vi "GetCellStrColor.vi"(7 "Color":u32, 8 "error in (no error)":errorcluster, 10 "Hdr Name":T1, 11 "Dynamic in":refnum<class "Dynamic.lvclass">) -> (0 "error out":errorcluster, 1 "Cell String":string, 2 "Cell Color":u32, 3 "Dynamic out":refnum<class "Dynamic.lvclass">)   [LabVIEW 2018, in "Measurement Channels.lvlib" / "Dynamic.lvclass"]
uses:
  Dynamic.lvclass
  Common/Controls/HeaderNames.ctl
  Dynamic.lvclass/Dynamic.ctl
  SubVIs Table/Custom Ctls Table/ge_ColType.ctl
  Class Voltage/Voltage.lvclass
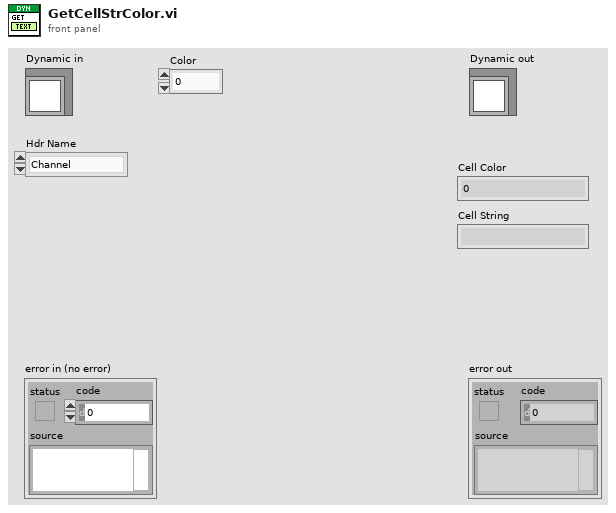
[diagram p1: front panel]
types:
  T1 = typedef "HeaderNames.ctl" = enum16{"Channel", "Device", "Spacer", "Description", "MB", "Range", "Terminal", "Coupling", "Thresh (V)", "Pulse/Rev", "Slope", "Min EU", "Min RPM", "mV/EU", "Iex", "Temp Units", "Type", "CJC Src", "CJC Val", "Ro", "Wire Cfg", "Strain Mode", "Vex", "Bridge Type", "GF", "Gauge Res", "Poisson", "Lead Res", "Init Strain", "GAF", "Scale", "Offset", "Unit (EU)", "dB?", "dB Ref", "Cal Mag", "Cal Units", "Max Temp", "Min Temp", "Max Strain", "Min Strain"}
  T2 = typedef "ge_ColType.ctl" = enum16{"Volts", "Amps", "Ohms", "TermCfg", "WireCfg", "Coup", "Slope", "Iex", "CalUnits", "ThrmUnits", "ThrmType", "CJCSrc", "BrdgType", "Strn Mode", "RTDType"}
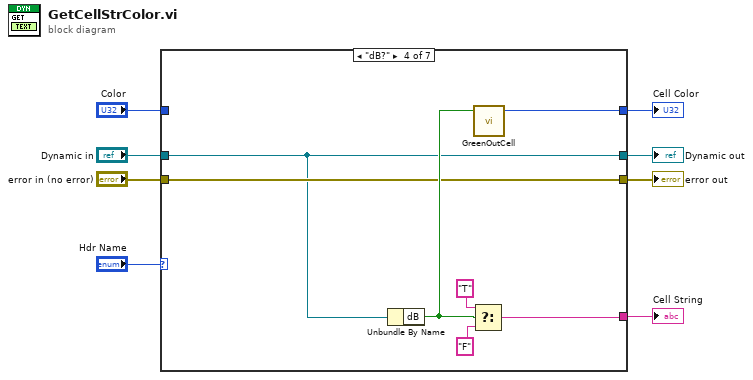
[diagram p0: block diagram]
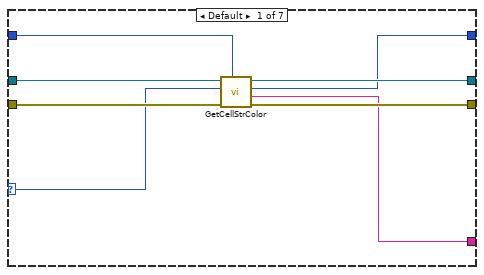
[diagram p2: hidden frame]
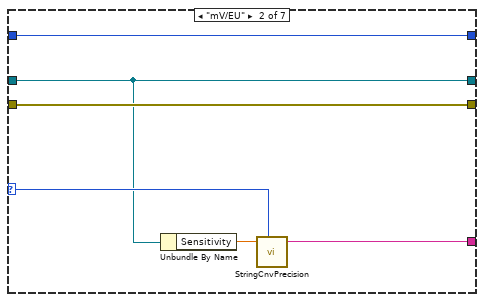
[diagram p3: hidden frame]
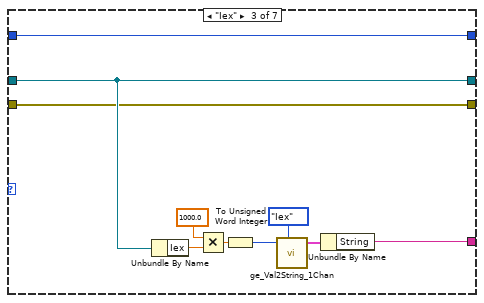
[diagram p4: hidden frame]
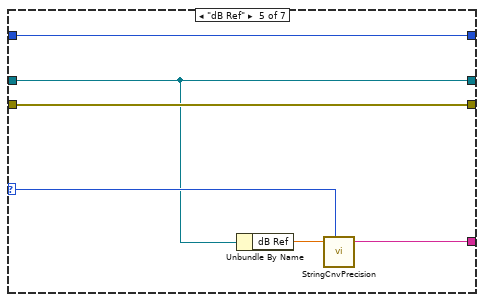
[diagram p5: hidden frame]
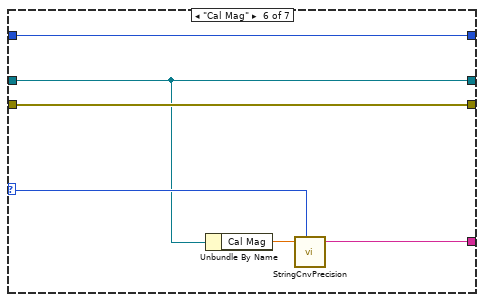
[diagram p6: hidden frame]
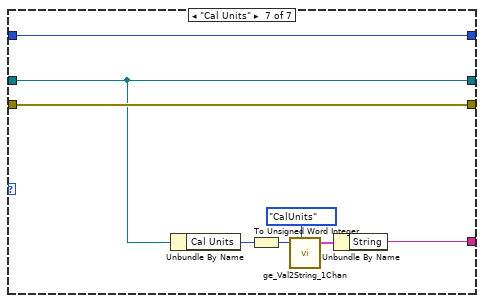
[diagram p7: hidden frame]
diagram:
  n1 = case shown="\"dB?\"" "Hdr Name" {
    selector: "Hdr Name" -> [w11 w19 _ _ w44 w50 _]
    tunnel: [w9 w18 w30 w37 w43 w49 w54] -> w1
    tunnel: [w10 w22 w23 w35 w40 w46 w59] -> w2
    tunnel: "Dynamic in" -> [w16 w17 w25 w33 w41 w47 w52]
    tunnel: [w15 w17 w25 w33 w41 w47 w52] -> w7
    tunnel: "error in (no error)" -> [w14 w21 w24 w34 w42 w48 w53]
    tunnel: [w13 w21 w24 w34 w42 w48 w53] -> w5
    tunnel: "Color" -> [w12 w22 w23 _ w40 w46 w59]
    frame Default {
      n2 = call-parent "GetCellStrColor.vi"("Color"=w12, "error in (no error)"=w14, "Hdr Name"=w11, "Voltage in"=w16) -> ("error out"=w13:errorcluster, "Cell String"=w9:string, "Cell Color"=w10:u32, "Voltage out"=w15:refnum<class "Dynamic.lvclass">)  [unwired: 4 in]
    }
    frame "mV/EU" {
      n3 = Unbundle By Name(w17) -> ("Sensitivity"=w20:dbl)
      n4 = call "StringCnvPrecision.vi"("Number"=w20, "Header"=w19) -> ("Float String"=w18:string)  [unwired: 5 in]
    }
    frame "Iex" {
      n5 = Unbundle By Name(w25) -> ("Iex"=w27:dbl)
      n6 = Multiply(x=1000.0, y=w27) -> (x*y=w29:dbl)
      n7 = To Unsigned Word Integer(number=w29) -> (unsigned 16bit integer=w26:u16)
      n8 = call "ge_Val2String_1Chan.vi"("Value"=w26, "ColType"=ge_ColType."Iex") -> ("String and Val"=w31:cluster{"String":string, "Value":u16})  [unwired: 5 in]
      n9 = Unbundle By Name(w31) -> ("String"=w30:string)
    }
    frame "dB?" {
      n10 = Unbundle By Name(w33) -> ("dB"=w36:bool)
      n11 = Select(t="T", s=w36, f="F") -> (s? t:f=w37:string)
      n12 = call "GreenOutCell.vi"("ToModBus?"=w36) -> ("Color"=w35:u32)  [unwired: 4 in]
    }
    frame "dB Ref" {
      n13 = Unbundle By Name(w41) -> ("dB Ref"=w45:dbl)
      n14 = call "StringCnvPrecision.vi"("Number"=w45, "Header"=w44) -> ("Float String"=w43:string)  [unwired: 5 in]
    }
    frame "Cal Mag" {
      n15 = Unbundle By Name(w47) -> ("Cal Mag"=w51:dbl)
      n16 = call "StringCnvPrecision.vi"("Number"=w51, "Header"=w50) -> ("Float String"=w49:string)  [unwired: 5 in]
    }
    frame "Cal Units" {
      n17 = Unbundle By Name(w52) -> ("Cal Units"=w55:u16)
      n18 = To Unsigned Word Integer(number=w55) -> (unsigned 16bit integer=w58:u16)
      n19 = call "ge_Val2String_1Chan.vi"("Value"=w58, "ColType"=ge_ColType."CalUnits") -> ("String and Val"=w56:cluster{"String":string, "Value":u16})  [unwired: 5 in]
      n20 = Unbundle By Name(w56) -> ("String"=w54:string)
    }
  }
  "error out" <- w5
  "Dynamic out" <- w7
  "Cell String" <- w1
  "Cell Color" <- w2
